vi "Motor Direction.vi"(10 "Backwards":bool, 11 "Forward":bool) -> (3 "Direction":dbl)   [LabVIEW 2014]
doc: "A boolean set motor controller for moving a motor forwards or backwards."
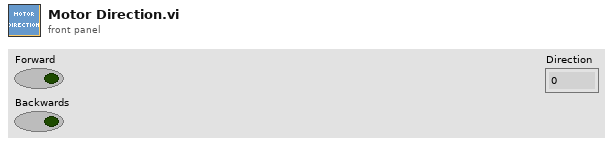
[diagram p1: front panel]
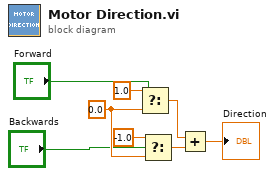
[diagram p0: block diagram]
diagram:
  w6 = 0.0
  n1 = Select(t=1.0, s="Forward", f=w6) -> (s? t:f=w5:dbl)
  n2 = Select(t=-1.0, s="Backwards", f=w6) -> (s? t:f=w4:dbl)
  n3 = Add(x=w5, y=w4) -> (x+y=→"Direction":dbl)
